vi "Set Prompt Message.vi"(0 "VISA resource name":refnum<visa-resource-name>, 5 "Prompt (empty)":string=" ", 11 "error in (no error)":errorcluster) -> (4 "VISA resource name out":refnum<visa-resource-name>, 15 "error out":errorcluster)   [LabVIEW 2020, in "Associated Research 78XX Series.lvlib"]
doc: "SP <prompt message>\nAdds or edits a prompt message for the active step."
uses:
  <instrlib>/Associated Research 78XX Series/Associated Research 78XX Series.lvlib
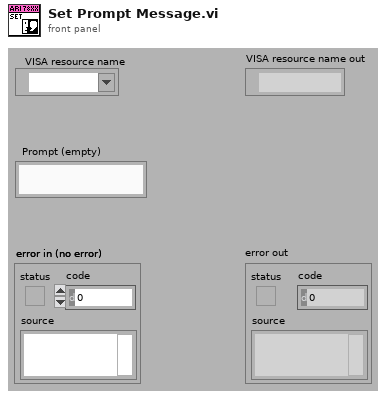
[diagram p1: front panel]
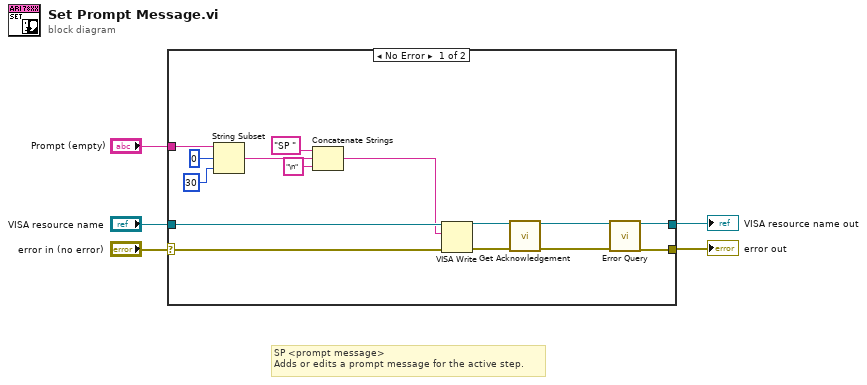
[diagram p0: block diagram]
diagram:
  # "SP <prompt message>\nAdds or edits a prompt message for the active step."
  n1 = case shown="No Error" "error in (no error)" {
    selector: "error in (no error)" -> [w11 w22]
    tunnel: "VISA resource name" -> [w20 w21]
    tunnel: [w19 w21] -> w4
    tunnel: [w18 w22] -> w3
    tunnel: "Prompt (empty)" -> [w12 _]
    frame No Error {
      n2 = String Subset(string=w12, offset (0)=0, length (rest)=30 ("length (rest)")) -> (substring=w17:string)
      n3 = Concatenate Strings("SP " ("\"False\" Command"), w17, "\n" ("string")) -> (w6:string)
      n4 = VISA Write(VISA resource name=w20, write buffer=w6, error in (no error)=w11) -> (VISA resource name out=w7:refnum<visa-resource-name>, error out=w8:errorcluster)  [unwired: 1 out]
      n5 = call <instrlib>:"Get Acknowledgement.vi"("VISA resource name"=w7, "error in (no error)"=w8) -> ("VISA resource name out"=w10:refnum<visa-resource-name>, "error out"=w9:errorcluster)  [unwired: 12 in]
      n6 = call <instrlib>:"Error Query.vi"("VISA resource name"=w10, "error in (no error)"=w9) -> ("VISA resource name out"=w19:refnum<visa-resource-name>, "error out"=w18:errorcluster)  [unwired: 10 in, 2 out]
    }
    frame Error {
    }
  }
  "error out" <- w3
  "VISA resource name out" <- w4
